vi "Decompose Cluster - Mixed - Element Value.vi"() -> ()   [LabVIEW 2017, in "Composition.Tests.lvlib"]
uses:
  Composition.Tests.lvlib
  Composition/Composition.lvlib
  <vilib>/addons/_JKI Toolkits/Caraya/classes/Test/Test.lvclass
  <vilib>/addons/_JKI Toolkits/Caraya/classes/Assert/Assert.lvclass
panel:
  out "error out":errorcluster
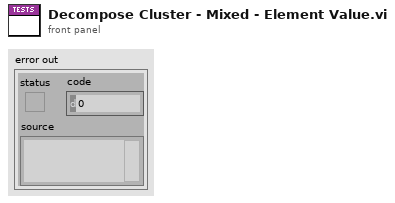
[diagram p1: front panel]
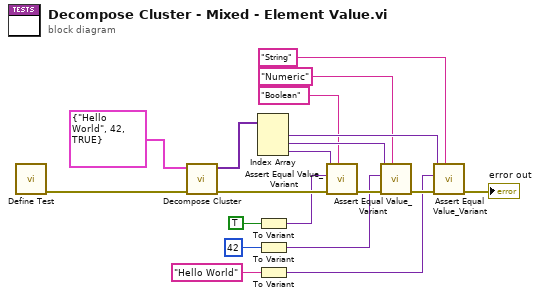
[diagram p0: block diagram]
diagram:
  n1 = call <vilib>:"Define Test.vi"() -> ("error out"=w10:errorcluster)  [unwired: 11 in]
  n2 = call "Decompose Cluster.vi"("error in (no error)"=w10, "Cluster"=cluster{string, i32, bool} {"Hello World", 42, TRUE}) -> ("error out"=w18:errorcluster, "Cluster Elements"=w16:variant[])  [unwired: 8 in]
  n3 = Index Array(array=w16) -> (element #1=w7:variant, element #2=w8:variant, element #3=w9:variant)  [unwired: 3 in]
  n4 = To Variant(anything=TRUE) -> (Variant=w6:variant)
  n5 = To Variant(anything=42) -> (Variant=w5:variant)
  n6 = To Variant(anything="Hello World") -> (Variant=w4:variant)
  n7 = call <vilib>:"Assert Equal Value_Variant.vi"("Label"="Boolean", "error in (no error)"=w18, "Y"=w6, "X"=w9) -> ("error out"=w17:errorcluster)  [unwired: 7 in]
  n8 = call <vilib>:"Assert Equal Value_Variant.vi"("Label"="Numeric", "error in (no error)"=w17, "Y"=w5, "X"=w8) -> ("error out"=w14:errorcluster)  [unwired: 7 in]
  n9 = call <vilib>:"Assert Equal Value_Variant.vi"("Label"="String", "error in (no error)"=w14, "Y"=w4, "X"=w7) -> ("error out"=→"error out":errorcluster)  [unwired: 7 in]
